vi "Sr830 Autoscale.vi"(4 "error in":errorcluster, 7 "Ressource VISA":refnum<visa-resource-name>="GPIB0::8::INSTR") -> (0 "error out":errorcluster, 1 "Sensitivity":u16(ring)=1 items=["2 nV/fA", "5 nV/fA", "10 nV/fA", "20 nV/fA", "50 nV/fA", "100 nV/fA", "200 nV/fA", "500 nV/fA", "1 µV/pA", "2 µV/pA", "5 µV/pA", "10 µV/pA", "20 µV/pA", "50 µV/pA", "100µV/pA", "200 µV/pA", "500µV/pA", "1 mV/nA", "2 mV/nA", "5 mV/nA", "10 mV/nA", "20 mV/nA", "50 mV/nA", "100 mV/nA", "200 mV/nA", "500 mV/nA", "1 V/uA"], 2 "OverRanged":bool, 3 "Ressource VISA Out":refnum<visa-resource-name>="GPIB0::8::INSTR")   [LabVIEW 2019]
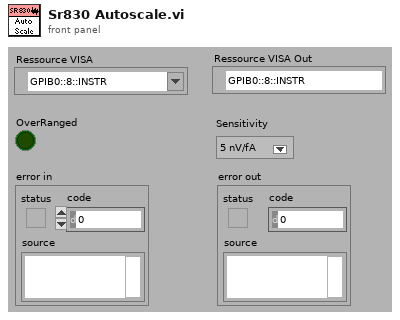
[diagram p1: front panel]
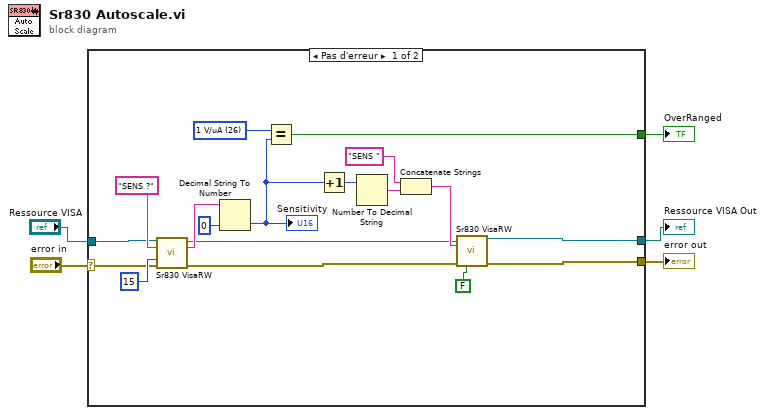
[diagram p0: block diagram]
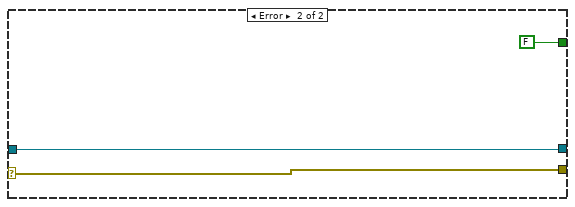
[diagram p2: hidden frame]
diagram:
  n1 = case shown="Pas d'erreur" "error in" {
    selector: "error in" -> [w18 w26]
    tunnel: [w9 w26] -> w5
    tunnel: [w11 FALSE] -> w4
    tunnel: "Ressource VISA" -> [w19 w24]
    tunnel: [w10 w24] -> w1
    frame No Error {
      w6 = u16 26 items=["2 nV/fA", "5 nV/fA", "10 nV/fA", "20 nV/fA", "50 nV/fA", "100 nV/fA", "200 nV/fA", "500 nV/fA", "1 µV/pA", "2 µV/pA", "5 µV/pA", "10 µV/pA", "20 µV/pA", "50 µV/pA", "100µV/pA", "200 µV/pA", "500µV/pA", "1 mV/nA", "2 mV/nA", "5 mV/nA", "10 mV/nA", "20 mV/nA", "50 mV/nA", "100 mV/nA", "200 mV/nA", "500 mV/nA", "1 V/uA"] ("Sensitivity")
      n2 = call <userlib>:"Sr830 VisaRW.vi"("VISA Rsrc"=w19, "ChaineCom"="SENS ?", "Nbcaract"=u32 15, "error in (no error)"=w18) -> ("VISA Rsrc Out"=w12:refnum<visa-resource-name>, "ChaineRep"=w21:string, "error out"=w13:errorcluster)  [unwired: 8 in, 1 out]
      n3 = Decimal String To Number(string=w21, default (0L)=u16 0 ("valeur par défaut (0 I32)")) -> (number=w7:u16)  [unwired: 1 in, 1 out]
      "Sensitivity" <- w7
      n4 = Equal?(x=w6, y=w7) -> (x = y?=w11:bool)
      n5 = Increment(x=w7) -> (x+1=w8:u16)
      n6 = Number To Decimal String(number=w8) -> (decimal integer string=w16:string)  [unwired: 1 in]
      n7 = Concatenate Strings("SENS " ("ChaineCom"), w16) -> (w14:string)
      n8 = call <userlib>:"Sr830 VisaRW.vi"("VISA Rsrc"=w12, "ChaineCom"=w14, "error in (no error)"=w13, "Lecture?(T)"=FALSE) -> ("VISA Rsrc Out"=w10:refnum<visa-resource-name>, "error out"=w9:errorcluster)  [unwired: 8 in, 2 out]
    }
    frame Error {
    }
  }
  "error out" <- w5
  "OverRanged" <- w4
  "Ressource VISA Out" <- w1
